vi "读取数据处理.vi"(10 "通讯读取数据":string) -> (1 "读取数据":i16[](array[numeric]), 2 "通讯状态":string)   [LabVIEW 2012]
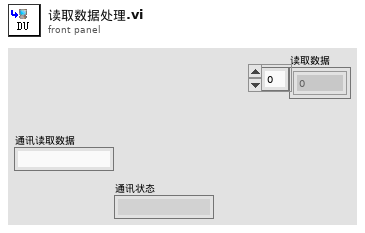
[diagram p1: front panel]
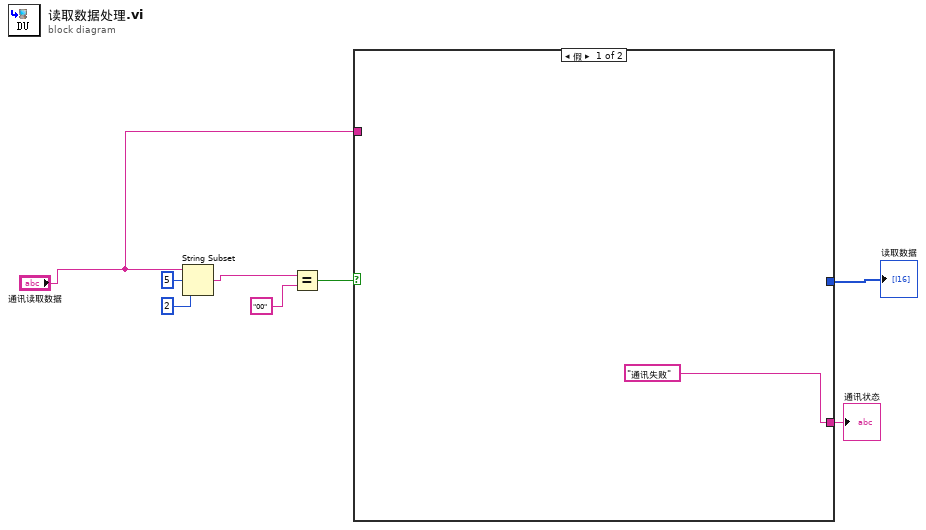
[diagram p0: block diagram]
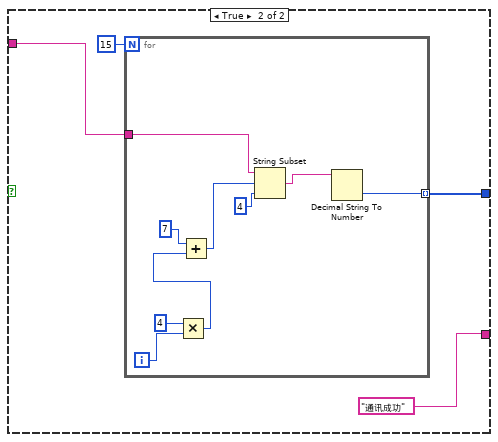
[diagram p2: hidden frame]
diagram:
  n1 = String Subset(string="通讯读取数据", offset (0)=5 ("偏移量(0)"), length (rest)=2 ("长度（剩余）")) -> (substring=w6:string)
  n2 = Equal?(x=w6, y="00") -> (x = y?=w4:bool)
  n3 = case shown="假" w4 {
    tunnel: "通讯读取数据" -> [_ w13]
    tunnel: [_ w11] -> w2
    tunnel: ["通讯失败" "通讯成功"] -> w1
    frame False {
    }
    frame True {
      n4 = for {
        N: 15 -> [_]
        tunnel: w13 -> [w16]
        tunnel: [w14] -> w11 mode=indexing
        i -> [w20]
        n5 = Multiply(x=4, y=w20) -> (x*y=w18:i32)
        n6 = Add(x=7 ("长度（剩余）"), y=w18) -> (x+y=w17:i32)
        n7 = String Subset(string=w16, offset (0)=w17, length (rest)=4 ("长度（剩余）")) -> (substring=w15:string)
        n8 = Decimal String To Number(string=w15) -> (number=w14:i32)  [unwired: 2 in, 1 out]
      }
    }
  }
  "读取数据" <- w2
  "通讯状态" <- w1
